vi "p_from_r.vi"(11 "r array in":dbl[](array[numeric])) -> (3 "P eff. out":dbl[](array[numeric]))   [LabVIEW 2018]
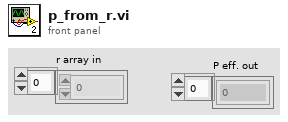
[diagram p1: front panel]
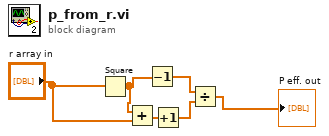
[diagram p0: block diagram]
diagram:
  n1 = Square(x="r array in") -> (x^2=w3:dbl[])
  n2 = Add(x=w3, y="r array in") -> (x+y=w5:dbl[])
  n3 = Decrement(x=w3) -> (x-1=w6:dbl[])
  n4 = Increment(x=w5) -> (x+1=w2:dbl[])
  n5 = Divide(x=w6, y=w2) -> (x/y=→"P eff. out":dbl[])
